vi "CanBurglerSol.vi"(8 "Error In":errorcluster, 11 "Grabber Open/Close":bool) -> (0 "Error Out":errorcluster)   [LabVIEW 2014]
uses:
  <vilib>/Rock Robotics/WPI/Solenoid/WPI_SolenoidValue.ctl
  Global Variables/Refnum Names.vi
  <vilib>/Rock Robotics/WPI/Solenoid/WPI_SolenoidSetEnum.vi
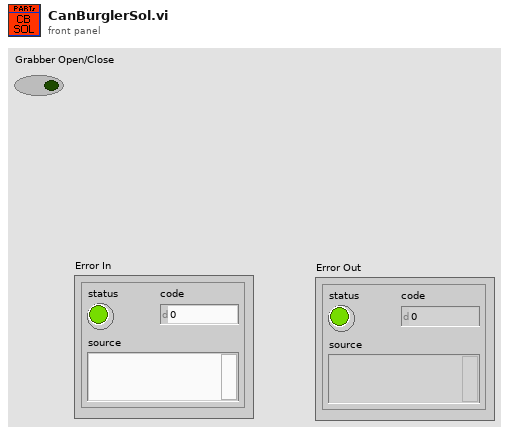
[diagram p1: front panel]
types:
  T1 = typedef "WPI_SolenoidValue.ctl" = enum16{"Off", "On", "Forward", "Reverse"}
  T2 = typedef "WPI_SolenoidDevRef.ctl" = cluster{"DevStatus":errorcluster, "Pneumatics Control Module":u8, "Forward Solenoid Channel":T3, "Reverse Solenoid Channel":T3}
  T3 = typedef "WPI_SolenoidChannel.ctl" = enum8{"Solenoid 0", "Solenoid 1", "Solenoid 2", "Solenoid 3", "Solenoid 4", "Solenoid 5", "Solenoid 6", "Solenoid 7", "Invalid"}
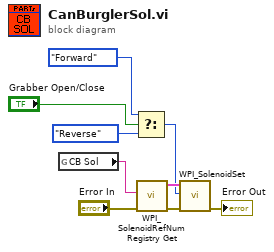
[diagram p0: block diagram]
diagram:
  n1 = global read "Refnum Names.vi" "CB Sol"() -> (w1:string)
  n2 = Select(t=WPI_SolenoidValue."Forward" ("Value"), s="Grabber Open/Close", f=WPI_SolenoidValue."Reverse" ("Value")) -> (s? t:f=w5:T1)
  n3 = call <vilib>:"WPI_SolenoidRefNum Registry Get.vi"("error in (no error)"="Error In", "refnum name"=w1) -> ("error out"=w7:errorcluster, "SolenoidDevRef"=w6:T2)  [unwired: 8 in]
  n4 = call-poly <vilib>:"WPI_SolenoidSet.vi"("error in (no error)"=w7, "Value"=w5, "SolenoidDevRef"=w6) -> ("error out"=→"Error Out":errorcluster)  [unwired: 7 in, 1 out]
